vi "Position PID servo.vi"(0 "FPGA VI Reference In":refnum<k20>, 1 "home offset cluster":T1, 2 "init offset cluster":T2, 5 "error in":errorcluster, 7 "command array":i32[](array[numeric]), 9 "L1 PID cluster":T6, 11 "L2 PID cluster":T5, 12 "L3 PID cluster":T4, 13 "L4 PID cluster":T3) -> (4 "FPGA VI Reference Out":refnum<k20>, 6 "error out":errorcluster)   [LabVIEW 2010]
doc: "This VI takes PID clusters, offsets and command array to go to a specific position using PID position servo."
uses:
  <vilib>/rvi/interface/nirviReadWriteControl/nirviReadWriteControl.xnode
  FPGA Bitfiles/IRISSControl_FPGATarget_IRISSFPGAIOv3.1_CU9txIsOgfM.lvbitx
  IRISS_FPGA_IO_v3.1.vi
panel:
  out "cmd L4":i32
  out "cmd L3":i32
  out "cmd L2":i32
  out "cmd L1":i32
  out "L4 init pos from home":i32 step=1111
  out "L3 init pos from home":i32 step=1111
  out "L2 init pos from home":i32 step=1111
  out "L1 init pos from home":i32 step=1111
  out "D L4":dbl=0.1
  out "L4 home offset":i32 step=1111
  out "L3 home offset":i32 step=1111
  out "L2 home offset":i32 step=1111
  out "L1 home offset":i32 step=1111
  out "Ave L3":i32=50
  out "I L3":dbl=0.0005
  out "D L3":dbl=1.0
  out "K L3":dbl=0.05
  out "Ave L2":i32=50
  out "I L2":dbl=0.0005
  out "D L2":dbl=1.0
  out "K L2":dbl=0.01
  out "Ave L1":i32=50
  out "K L1":dbl=0.005
  out "D L1":dbl=0.5
  out "I L1":dbl=0.0005
  out "Ave L4":i32=50
  out "I L4":dbl=0.0005
  out "K L4":dbl=0.1
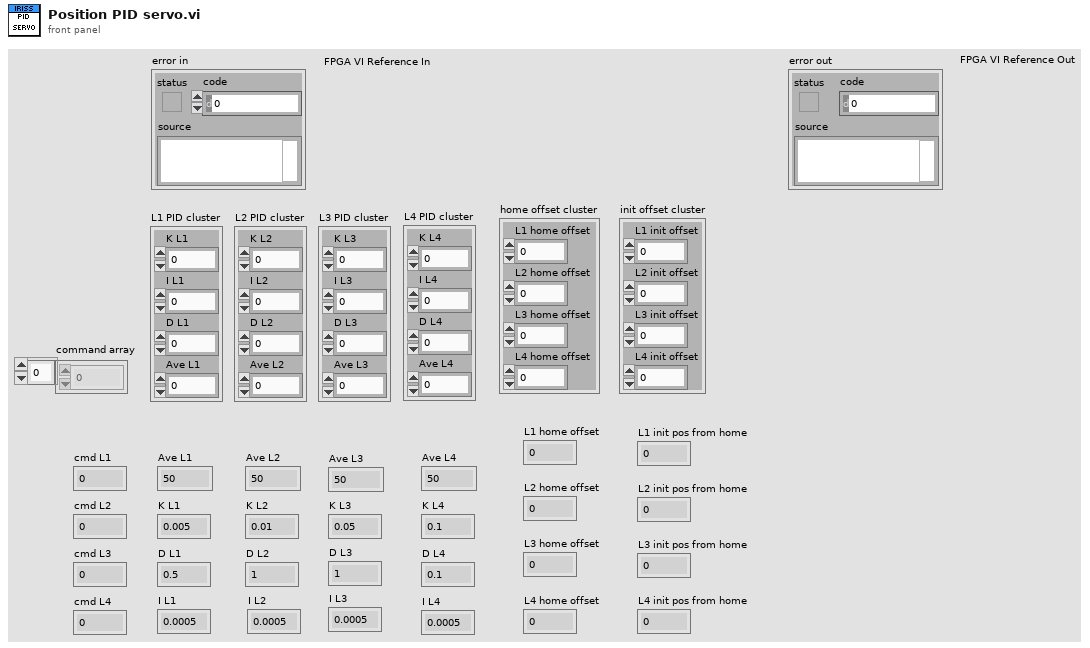
[diagram p1: front panel]
types:
  T1 = cluster{"L1 home offset":i32, "L2 home offset":i32, "L3 home offset":i32, "L4 home offset":i32}
  T2 = cluster{"L1 init offset":i32, "L2 init offset":i32, "L3 init offset":i32, "L4 init offset":i32}
  T3 = cluster{"K L4":dbl, "I L4":dbl, "D L4":dbl, "Ave L4":i32}
  T4 = cluster{"K L3":dbl, "I L3":dbl, "D L3":dbl, "Ave L3":i32}
  T5 = cluster{"K L2":dbl, "I L2":dbl, "D L2":dbl, "Ave L2":i32}
  T6 = cluster{"K L1":dbl, "I L1":dbl, "D L1":dbl, "Ave L1":i32}
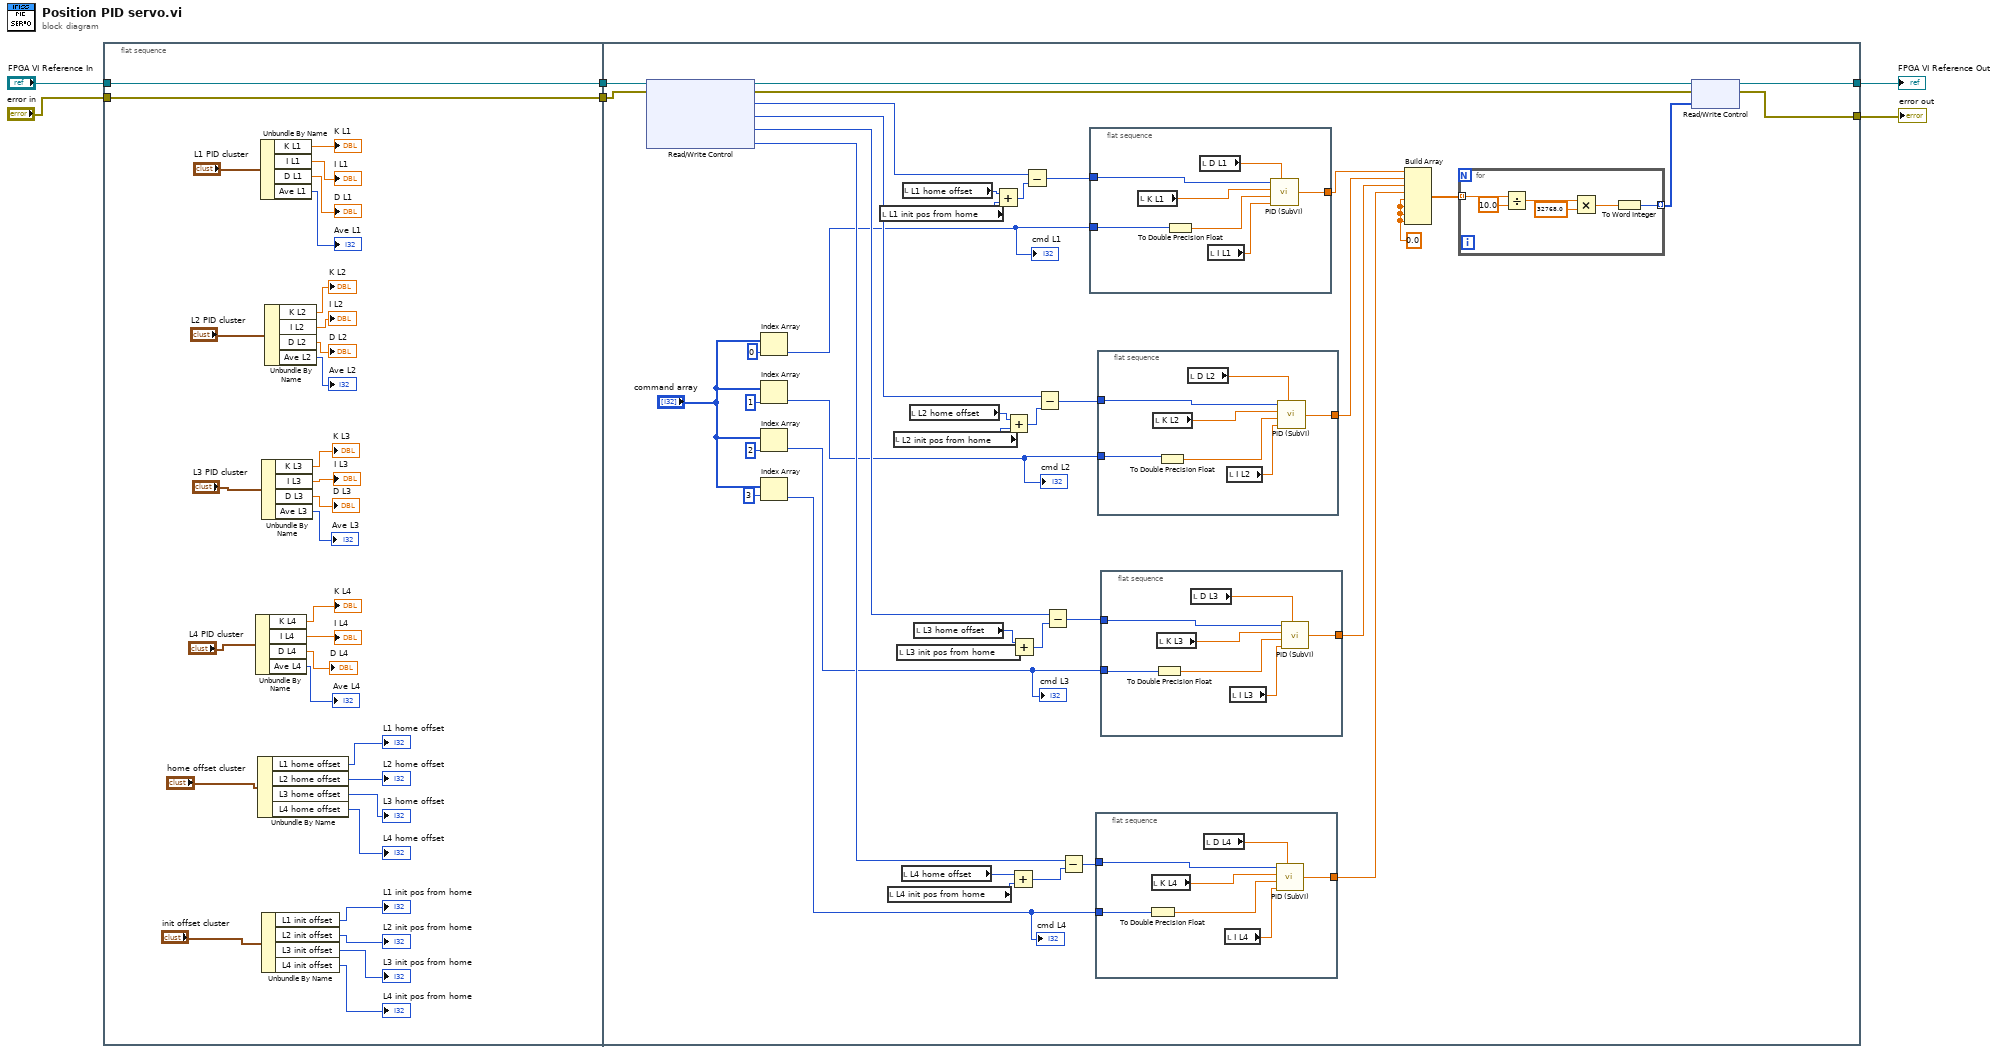
[diagram p0: block diagram]
diagram:
  n1 = flat-sequence {
    tunnel: [w38] -> w6
    tunnel: "FPGA VI Reference In" -> [w38]
    tunnel: [w37] -> w4
    tunnel: "error in" -> [w37]
    tunnel: w6 -> [w51]
    tunnel: w4 -> [w50]
    tunnel: [w49] -> w1
    tunnel: [w48] -> w2
    frame #0 {
      n2 = Unbundle By Name("L4 PID cluster") -> ("K L4"=→"K L4":dbl, "I L4"=→"I L4":dbl, "D L4"=→"D L4":dbl, "Ave L4"=→"Ave L4":i32)
      n3 = Unbundle By Name("home offset cluster") -> ("L1 home offset"=→"L1 home offset":i32, "L2 home offset"=→"L2 home offset":i32, "L3 home offset"=→"L3 home offset":i32, "L4 home offset"=→"L4 home offset":i32)
      n4 = Unbundle By Name("L1 PID cluster") -> ("K L1"=→"K L1":dbl, "I L1"=→"I L1":dbl, "D L1"=→"D L1":dbl, "Ave L1"=→"Ave L1":i32)
      n5 = Unbundle By Name("L3 PID cluster") -> ("K L3"=→"K L3":dbl, "I L3"=→"I L3":dbl, "D L3"=→"D L3":dbl, "Ave L3"=→"Ave L3":i32)
      n6 = Unbundle By Name("init offset cluster") -> ("L1 init offset"=→"L1 init pos from home":i32, "L2 init offset"=→"L2 init pos from home":i32, "L3 init offset"=→"L3 init pos from home":i32, "L4 init offset"=→"L4 init pos from home":i32)
      n7 = Unbundle By Name("L2 PID cluster") -> ("K L2"=→"K L2":dbl, "I L2"=→"I L2":dbl, "D L2"=→"D L2":dbl, "Ave L2"=→"Ave L2":i32)
    }
    frame #1 {
      w80 = 0.0 ("element")
      n8 = xnode "Read/Write Control"("FPGA VI Reference In"=w51, "error in"=w50) -> ("FPGA VI Reference Out"=w77:refnum<k20>, "error out"=w76:errorcluster, "32 bit Position 1"=w63:i32, "32 bit Position 3"=w62:i32, "32 bit Position C1-1"=w57:i32, "32 bit Position C1-4"=w56:i32)
      n9 = Index Array(array="command array", index=0) -> (element=w42:i32)
      "cmd L1" <- w42
      n10 = Index Array(array="command array", index=1) -> (element=w41:i32)
      "cmd L2" <- w41
      n11 = Index Array(array="command array", index=2) -> (element=w40:i32)
      "cmd L3" <- w40
      n12 = Index Array(array="command array", index=3) -> (element=w39:i32)
      "cmd L4" <- w39
      n13 = local read "L1 init pos from home"() -> (w55:i32)
      n14 = local read "L4 init pos from home"() -> (w52:i32)
      n15 = local read "L2 init pos from home"() -> (w54:i32)
      n16 = local read "L3 init pos from home"() -> (w53:i32)
      n17 = local read "L4 home offset"() -> (w60:i32)
      n18 = local read "L1 home offset"() -> (w70:i32)
      n19 = local read "L2 home offset"() -> (w67:i32)
      n20 = local read "L3 home offset"() -> (w64:i32)
      n21 = Add(x=w70, y=w55) -> (x+y=w71:i32)
      n22 = Add(x=w67, y=w54) -> (x+y=w68:i32)
      n23 = Add(x=w60, y=w52) -> (x+y=w61:i32)
      n24 = Add(x=w64, y=w53) -> (x+y=w65:i32)
      n25 = Subtract(x=w63, y=w71) -> (x-y=w69:i32)
      n26 = Subtract(x=w62, y=w68) -> (x-y=w66:i32)
      n27 = Subtract(x=w57, y=w65) -> (x-y=w58:i32)
      n28 = Subtract(x=w56, y=w61) -> (x-y=w59:i32)
      n29 = flat-sequence {
        tunnel: w69 -> [w100]
        tunnel: [w99] -> w75
        tunnel: w42 -> [w94]
        frame #0 {
          n30 = local read "K L1"() -> (w96:dbl)
          n31 = To Double Precision Float(number=w94) -> (double precision float=w95:dbl)
          n32 = local read "D L1"() -> (w98:dbl)
          n33 = local read "I L1"() -> (w97:dbl)
          n34 = call "PID (SubVI).vi"("Feedback"=w100, "K"=w96, "Reference"=w95, "I"=w97, "D"=w98) -> ("Control Out"=w99:dbl)
        }
      }
      n35 = flat-sequence {
        tunnel: w59 -> [w93]
        tunnel: [w90] -> w72
        tunnel: w39 -> [w88]
        frame #0 {
          n36 = To Double Precision Float(number=w88) -> (double precision float=w87:dbl)
          n37 = local read "K L4"() -> (w92:dbl)
          n38 = local read "D L4"() -> (w89:dbl)
          n39 = local read "I L4"() -> (w91:dbl)
          n40 = call "PID (SubVI).vi"("Feedback"=w93, "K"=w92, "Reference"=w87, "I"=w91, "D"=w89) -> ("Control Out"=w90:dbl)
        }
      }
      n41 = flat-sequence {
        tunnel: w66 -> [w107]
        tunnel: [w103] -> w74
        tunnel: w41 -> [w102]
        frame #0 {
          n42 = local read "K L2"() -> (w105:dbl)
          n43 = To Double Precision Float(number=w102) -> (double precision float=w101:dbl)
          n44 = local read "D L2"() -> (w106:dbl)
          n45 = local read "I L2"() -> (w104:dbl)
          n46 = call "PID (SubVI).vi"("Feedback"=w107, "K"=w105, "Reference"=w101, "I"=w104, "D"=w106) -> ("Control Out"=w103:dbl)
        }
      }
      n47 = flat-sequence {
        tunnel: w58 -> [w114]
        tunnel: [w110] -> w73
        tunnel: w40 -> [w109]
        frame #0 {
          n48 = To Double Precision Float(number=w109) -> (double precision float=w108:dbl)
          n49 = local read "K L3"() -> (w112:dbl)
          n50 = local read "D L3"() -> (w113:dbl)
          n51 = local read "I L3"() -> (w111:dbl)
          n52 = call "PID (SubVI).vi"("Feedback"=w114, "K"=w112, "Reference"=w108, "I"=w111, "D"=w113) -> ("Control Out"=w110:dbl)
        }
      }
      n53 = Build Array(w75, w74, w73, w72, w80, w80, w80, w80) -> (w78:dbl[])
      n54 = for {
        tunnel: [w84] -> w79 mode=indexing
        tunnel: w78 -> [w83] mode=indexing
        n55 = Divide(x=w83, y=10.0) -> (x/y=w86:dbl)
        n56 = Multiply(x=w86, y=32768.0) -> (x*y=w85:dbl)
        n57 = To Word Integer(number=w85) -> (16bit integer=w84:i16)
      }
      n58 = xnode "Read/Write Control"("FPGA VI Reference In"=w77, "error in"=w76, "AO"=w79) -> ("FPGA VI Reference Out"=w49:refnum<k20>, "error out"=w48:errorcluster)
    }
  }
  "FPGA VI Reference Out" <- w1
  "error out" <- w2
